vi "ImageUpdateImage-2D.vi"(8 "error in (no error)":errorcluster, 11 "Image in":refnum<class "Image.lvclass">) -> (0 "error out":errorcluster, 1 "Images Displayed":i32, 3 "Image out":refnum<class "Image.lvclass">)   [LabVIEW 2012, in "Image.lvclass"]
uses:
  classes/Image.lvclass
  classes/Image.lvclass/Image.ctl
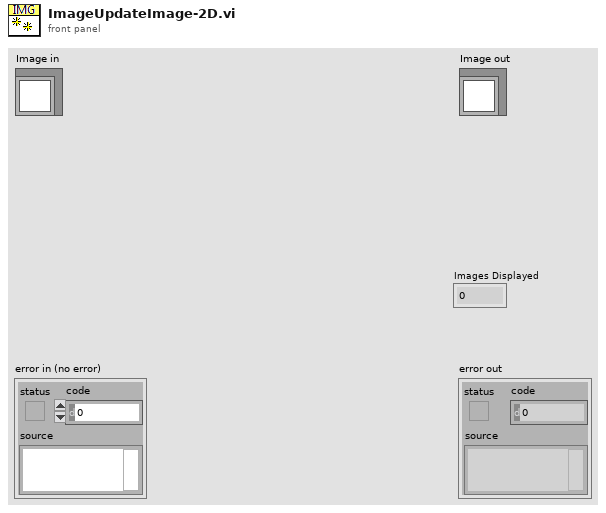
[diagram p1: front panel]
types:
  T1 = typedef "Scan Type.ctl" = enum16{"None", "Point", "Full Image Continuous", "Full Image Grab"}
  T2 = typedef "Move Type.ctl" = enum16{"None", "Continuous", "Discrete"}
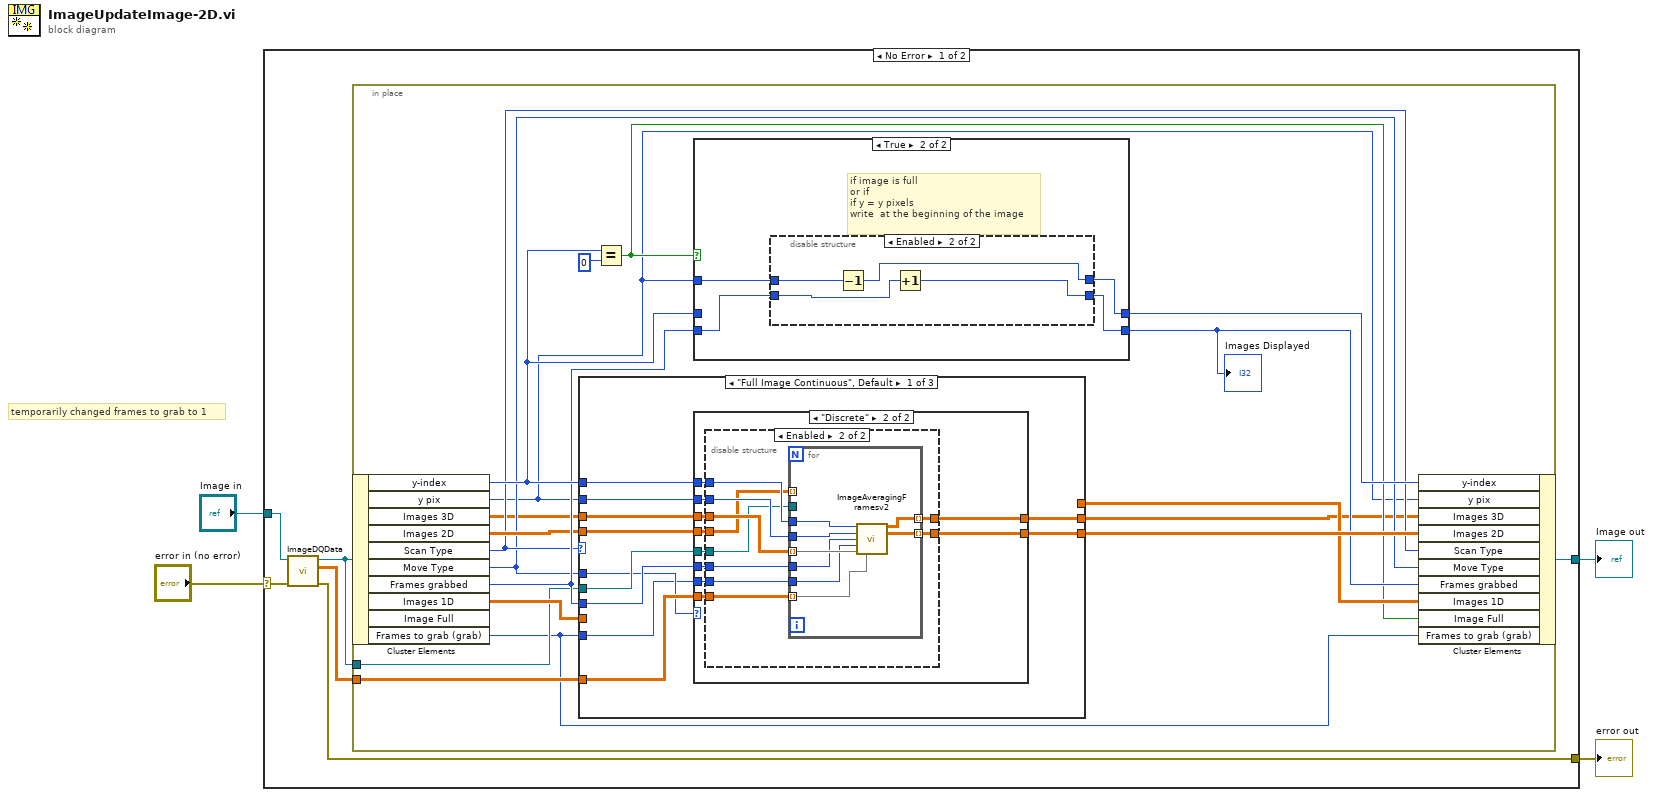
[diagram p0: block diagram]
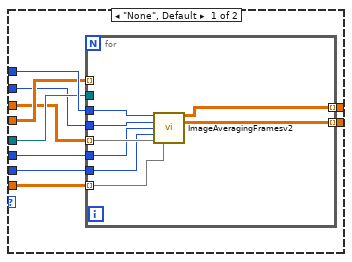
[diagram p2: hidden frame]
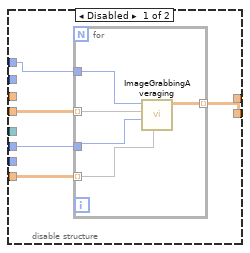
[diagram p3: hidden frame]
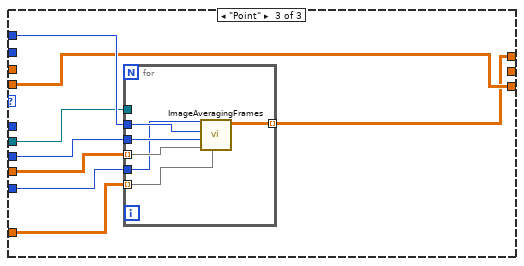
[diagram p5: hidden frame]
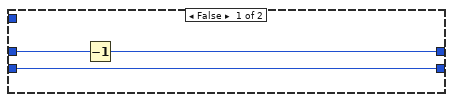
[diagram p6: hidden frame]
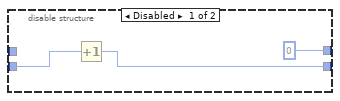
[diagram p7: hidden frame]
diagram:
  # "temporarily changed frames to grab to 1"
  n1 = case shown="No Error" "error in (no error)" {
    selector: "error in (no error)" -> [w6 w125]
    tunnel: [w5 w125] -> w3
    tunnel: [w10 w124] -> w2
    tunnel: "Image in" -> [w7 w124]
    frame No Error {
      n2 = call "ImageDQData.vi"("error in (no error)"=w6, "Image in"=w7) -> ("error out"=w5:errorcluster, "data"=w8:dbl[][], "Image out"=w9:refnum<class "Image.lvclass">)  [unwired: 7 in]
      n3 = in-place {
        in-place-border: w8 -> [w23]
        in-place-border: w9 -> [w20]
        n4 = in-place-cluster #1(w9) -> ("y-index"=w27:i32, "y pix"=w12:i32, "Images 3D"=w15:dbl[][][][], "Images 2D"=w24:dbl[][][], "Scan Type"=w17:T1, "Move Type"=w16:T2, "Frames grabbed"=w26:i32, "Images 1D"=w21:dbl[][][], "Frames to grab (grab)"=w11:i32)  [unwired: 1 out]
        n5 = case shown="\"Full Image Continuous\", Default" w17 {
          tunnel: w27 -> [w39 _ w103]
          tunnel: w24 -> [w38 _ w102]
          tunnel: w26 -> [w37 _ w101]
          tunnel: w20 -> [w36 _ w97]
          tunnel: [w33 _ w102] -> w25
          tunnel: w23 -> [w35 _ w100]
          tunnel: [_ _ w98] -> w22
          tunnel: w21 -> [_ _ w99]
          tunnel: w16 -> [w34 _ _]
          tunnel: w15 -> [w32 _ _]
          tunnel: [w31 _ _] -> w14
          tunnel: w11 -> [w30 _ w96]
          tunnel: w12 -> [w29 _ _]
          frame "Full Image Continuous", Default {
            n6 = case shown="\"Discrete\"" w34 {
              tunnel: w39 -> [w49 w66]
              tunnel: w38 -> [w48 w65]
              tunnel: w37 -> [w47 w64]
              tunnel: w36 -> [w46 w60]
              tunnel: [w45 w67] -> w33
              tunnel: w35 -> [w44 w63]
              tunnel: w32 -> [w43 w61]
              tunnel: [w42 w58] -> w31
              tunnel: w30 -> [w41 w59]
              tunnel: w29 -> [w40 w62]
              frame "None", Default {
                n7 = for {
                  tunnel: w49 -> [w53]
                  tunnel: w48 -> [_] mode=indexing
                  tunnel: w47 -> [w51]
                  tunnel: w46 -> [_]
                  tunnel: [w56] -> w45 mode=indexing
                  tunnel: w44 -> [w57] mode=indexing
                  tunnel: w43 -> [w54] mode=indexing
                  tunnel: [w55] -> w42 mode=indexing
                  tunnel: w41 -> [w50]
                  tunnel: w40 -> [w52]
                  n8 = call "ImageAveragingFramesv2.vi"("y-index"=w53, "x pix"=w52, "Frames grabbed"=w51, "Frames to grab (grab)"=w50, "Images 3D in"=w54, "new"=w57) -> ("Images 3D out"=w55:dbl[][][], "Images 2D out"=w56:dbl[][])  [unwired: 8 in]
                }
              }
              frame "Discrete" {
                n9 = disable-structure shown="Enabled" {
                  disable-tunnel: [w72 w78] -> w67
                  disable-tunnel: w66 -> [w71 w87]
                  disable-tunnel: w65 -> [w70 w84]
                  disable-tunnel: w64 -> [w69 w82]
                  disable-tunnel: w63 -> [w68 w80]
                  disable-tunnel: w62 -> [_ w86]
                  disable-tunnel: w61 -> [_ w85]
                  disable-tunnel: w60 -> [_ w83]
                  disable-tunnel: w59 -> [_ w81]
                  disable-tunnel: [_ w79] -> w58
                  frame Disabled {
                    n10 = for {
                      tunnel: [w77] -> w72 mode=indexing
                      tunnel: w71 -> [w76]
                      tunnel: w70 -> [w75] mode=indexing
                      tunnel: w69 -> [w74]
                      tunnel: w68 -> [w73] mode=indexing
                      n11 = call "ImageGrabbingAveraging.vi"("new"=w73, "Frames grabbed"=w74, "Images 2D in"=w75, "y-index"=w76) -> ("Images 2D out"=w77:dbl[][])  [unwired: 7 in]
                    }
                  }
                  frame Enabled {
                    n12 = for {
                      tunnel: w87 -> [w91]
                      tunnel: w84 -> [_] mode=indexing
                      tunnel: w82 -> [w89]
                      tunnel: w83 -> [_]
                      tunnel: [w94] -> w78 mode=indexing
                      tunnel: w80 -> [w95] mode=indexing
                      tunnel: w85 -> [w92] mode=indexing
                      tunnel: [w93] -> w79 mode=indexing
                      tunnel: w81 -> [w88]
                      tunnel: w86 -> [w90]
                      n13 = call "ImageAveragingFramesv2.vi"("y-index"=w91, "x pix"=w90, "Frames grabbed"=w89, "Frames to grab (grab)"=w88, "Images 3D in"=w92, "new"=w95) -> ("Images 3D out"=w93:dbl[][][], "Images 2D out"=w94:dbl[][])  [unwired: 8 in]
                    }
                  }
                }
              }
            }
          }
          frame "None" {
          }
          frame "Point" {
            n14 = for {
              tunnel: w103 -> [w106]
              tunnel: w99 -> [w107] mode=indexing
              tunnel: w101 -> [w105]
              tunnel: w97 -> [_]
              tunnel: [w108] -> w98 mode=indexing
              tunnel: w100 -> [w109] mode=indexing
              tunnel: w96 -> [w104]
              n15 = call "ImageAveragingFrames.vi"("new"=w109, "Images 2D in"=w107, "Frames grabbed"=w105, "y-index"=w106, "Frames to Grab"=w104) -> ("Images 2D out"=w108:dbl[][])  [unwired: 6 in]
            }
          }
        }
        n16 = Equal?(x=w27, y=0) -> (x = y?=w18:bool)
        n17 = case shown="True" w18 {
          tunnel: w27 -> [w111 _]
          tunnel: [w112 w114] -> w28
          tunnel: [w110 w116] -> w19
          tunnel: w26 -> [w110 w115]
          tunnel: w12 -> [_ w113]
          frame False {
            n18 = Decrement(x=w111) -> (x-1=w112:i32)
          }
          frame True {
            # "if image is full\nor if\nif y = y pixels\nwrite  at the beginning of the image"
            n19 = disable-structure shown="Enabled" {
              disable-tunnel: [w119 w123] -> w116
              disable-tunnel: w115 -> [w118 w122]
              disable-tunnel: [0 ("t") w120] -> w114
              disable-tunnel: w113 -> [_ w121]
              frame Disabled {
                n20 = Increment(x=w118) -> (x+1=w119:i32)
              }
              frame Enabled {
                n21 = Decrement(x=w121) -> (x-1=w120:i32)
                n22 = Increment(x=w122) -> (x+1=w123:i32)
              }
            }
          }
        }
        "Images Displayed" <- w19
        n23 = in-place-cluster #1("y-index"=w28, "y pix"=w12, "Images 3D"=w14, "Images 2D"=w25, "Scan Type"=w17, "Move Type"=w16, "Frames grabbed"=w19, "Images 1D"=w22, "Image Full"=w18, "Frames to grab (grab)"=w11) -> (w10:refnum<class "Image.lvclass">)
      }
    }
    frame Error {
    }
  }
  "error out" <- w3
  "Image out" <- w2
